vi "SwerveDriveSetSensorOffset.vi"(4 "Front Right Left Offset":dbl, 6 "Front Left Offset":dbl, 8 "error in (no error)":errorcluster, 9 "Rear Right Offset":dbl, 10 "Rear Left Offset":dbl, 11 "SwerveDriveDevRef":T1={"DevStatus"={"status"=FALSE, "code"=0, "source"=""}, "TurnMotors[]"=[], "Square Inputs"=FALSE, "Max Output"=1.0, "DriveMotors[]"=[], "WheelOffset[]"=[], "SwerveSensors[]"=[], "RobotSize"={"Width"=[], "Length"=[], "Center"=[]}}) -> (0 "error out":errorcluster, 3 "SwerveDriveDevRef":T1={"DevStatus"={"status"=FALSE, "code"=0, "source"=""}, "TurnMotors[]"=[], "Square Inputs"=FALSE, "Max Output"=1.0, "DriveMotors[]"=[], "WheelOffset[]"=[], "SwerveSensors[]"=[], "RobotSize"={"Width"=[], "Length"=[], "Center"=[]}})   [LabVIEW 2019, in "Swerve Drive.lvlib"]
uses:
  Swerve Drive.lvlib
  SwerveDriveDevRef.ctl
  <vilib>/Rock Robotics/WPI/MotorControl/WPI_MotorControlDeviceRef.ctl
  <vilib>/Rock Robotics/WPI/MotorControl/WPI_MotorControlType.ctl
  <vilib>/Rock Robotics/SystemInterfaces/DIO/FPGA_DIOPWMChannel.ctl
  <vilib>/Rock Robotics/WPI/PWM/WPI_PWMDeadband.ctl
  <vilib>/Rock Robotics/SystemInterfaces/DIO/FPGA_DIOChannel.ctl
  <vilib>/Rock Robotics/SystemInterfaces/AI/FPGA_AIChannel.ctl
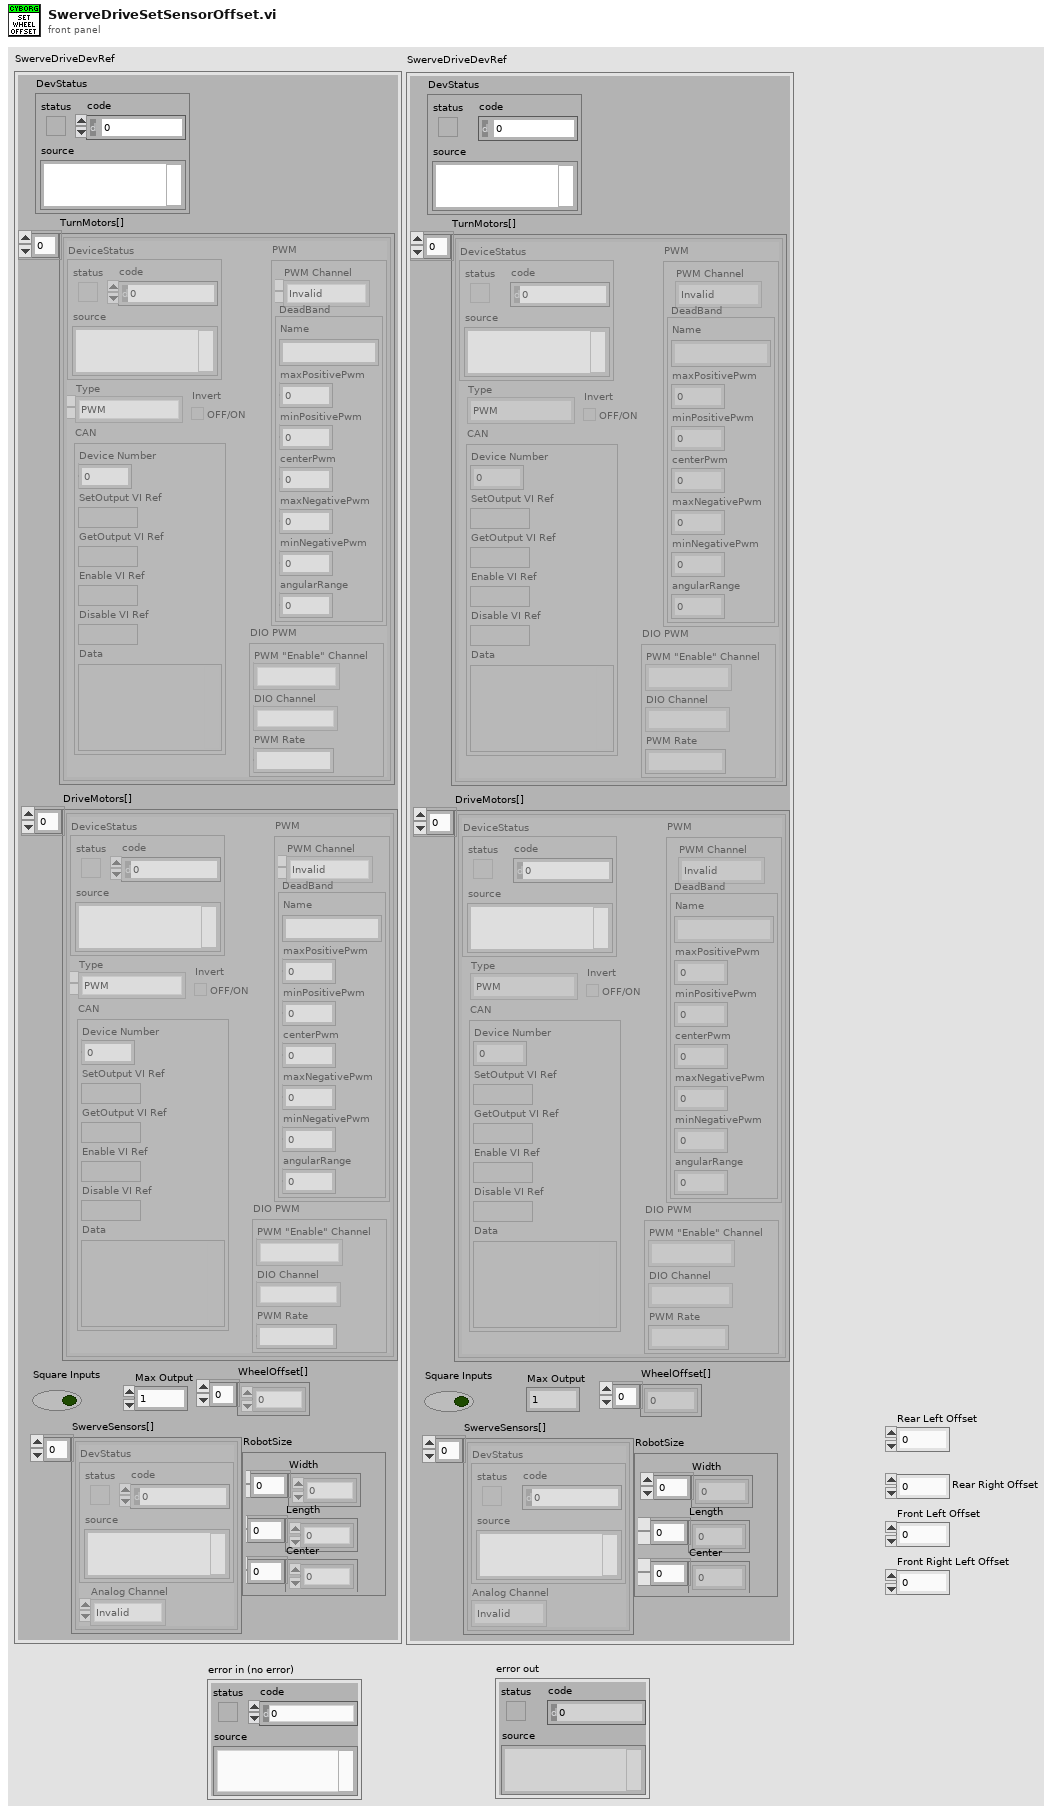
[diagram p1: front panel]
types:
  T1 = typedef "Swerve Drive.lvlib/SwerveDriveDevRef.ctl" = cluster{"DevStatus":errorcluster, "TurnMotors[]":T2[], "Square Inputs":bool, "Max Output":dbl, "DriveMotors[]":T2[], "WheelOffset[]":dbl[], "SwerveSensors[]":cluster{"DevStatus":errorcluster, "Analog Channel":T7}[], "RobotSize":cluster{"Width":dbl[], "Length":dbl[], "Center":dbl[]}}
  T2 = typedef "WPI_MotorControlDeviceRef.ctl" = cluster{"DeviceStatus":errorcluster, "Type":T3, "PWM":cluster{"PWM Channel":T4, "DeadBand":T5}, "CAN":cluster{"Device Number":u8, "SetOutput VI Ref":variant, "GetOutput VI Ref":variant, "Enable VI Ref":variant, "Disable VI Ref":variant, "Data":variant}, "Invert":bool, "DIO PWM":cluster{"PWM \"Enable\" Channel":T4, "DIOChannel":T6, "PWM Rate":dbl}}
  T3 = typedef "WPI_MotorControlType.ctl" = enum16{"PWM", "CAN", "DIO PWM"}
  T4 = typedef "FPGA_DIOPWMChannel.ctl" = enum8{"PWM 0", "PWM 1", "PWM 2", "PWM 3", "PWM 4", "PWM 5", "PWM 6", "PWM 7", "PWM 8", "PWM 9", "PWM MXP 0", "PWM MXP 1", "PWM MXP 2", "PWM MXP 3", "PWM MXP 4", "PWM MXP 5", "PWM MXP 6", "PWM MXP 7", "PWM MXP 8", "PWM MXP 9", "Invalid"}
  T5 = typedef "WPI_PWMDeadband.ctl" = cluster{"Name":string, "maxPositivePwm":i32, "minPositivePwm":i32, "centerPwm":i32, "maxNegativePwm":i32, "minNegativePwm":i32, "angularRange":u16}
  T6 = typedef "FPGA_DIOChannel.ctl" = enum8{"DIO 0", "DIO 1", "DIO 2", "DIO 3", "DIO 4", "DIO 5", "DIO 6", "DIO 7", "DIO 8", "DIO 9", "DIO MXP 0", "DIO MXP 1", "DIO MXP 2", "DIO MXP 3", "DIO MXP 4", "DIO MXP 5", "DIO MXP 6", "DIO MXP 7", "DIO MXP 8", "DIO MXP 9", "DIO MXP 10", "DIO MXP 11", "DIO MXP 12", "DIO MXP 13", "DIO MXP 14", "DIO MXP 15", "SPI Port CS1", "SPI Port CS2", "SPI Port CS3", "SPI Port MISO", "SPI Port MOSI", "Invalid"}
  T7 = typedef "FPGA_AIChannel.ctl" = enum8{"AI 0", "AI 1", "AI 2", "AI 3", "AI MXP 0", "AI MXP 1", "AI MXP 2", "AI MXP 3", "Invalid"}
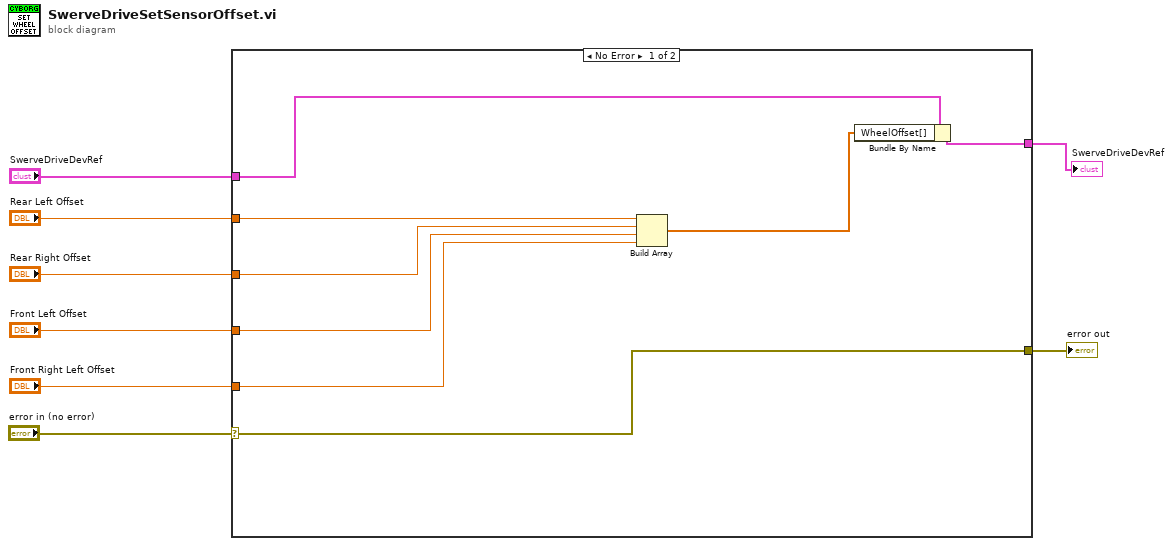
[diagram p0: block diagram]
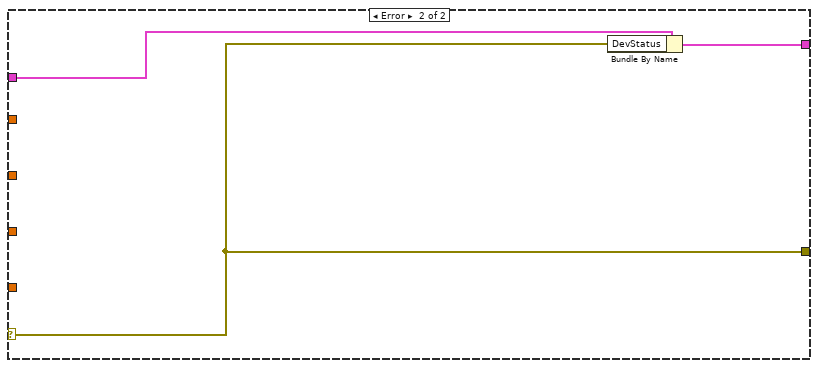
[diagram p2: hidden frame]
diagram:
  n1 = case shown="No Error" "error in (no error)" {
    selector: "error in (no error)" -> [w16 w17]
    tunnel: [w16 w17] -> w7
    tunnel: "SwerveDriveDevRef" -> [w14 w19]
    tunnel: [w15 w18] -> w5
    tunnel: "Rear Left Offset" -> [w13 _]
    tunnel: "Rear Right Offset" -> [w12 _]
    tunnel: "Front Left Offset" -> [w11 _]
    tunnel: "Front Right Left Offset" -> [w10 _]
    frame No Error {
      n2 = Build Array(w13, w12, w11, w10) -> (w9:dbl[])
      n3 = Bundle By Name(cluster=w14, "WheelOffset[]"=w9) -> (w15:T1)
    }
    frame Error {
      n4 = Bundle By Name(cluster=w19, "DevStatus"=w17) -> (w18:T1)
    }
  }
  "SwerveDriveDevRef" <- w5
  "error out" <- w7
